vi "Check Admin Identity.vi"(8 "error in (no error)":errorcluster, 10 "UserName(\"\")":string, 11 "User_Actor in":refnum<class "User_Actor.lvclass">) -> (0 "error out":errorcluster, 2 "Identity（False）":bool, 3 "User_Actor out":refnum<class "User_Actor.lvclass">)   [LabVIEW 2015, in "User_Actor.lvlib" / "User_Actor.lvclass"]
uses:
  User_Actor.lvclass
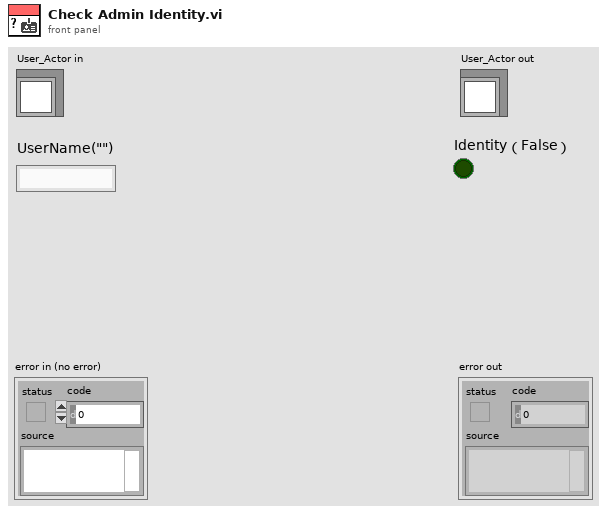
[diagram p1: front panel]
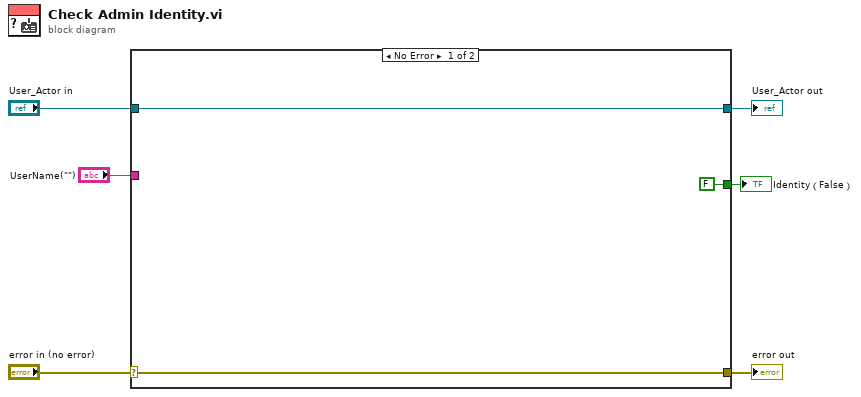
[diagram p0: block diagram]
diagram:
  n1 = case shown="No Error" "error in (no error)" {
    selector: "error in (no error)" -> [w9 w11]
    tunnel: [w9 w11] -> w5
    tunnel: [w8 w10] -> w3
    tunnel: "User_Actor in" -> [w8 w10]
    tunnel: "UserName(\"\")" -> [_ _]
    tunnel: [FALSE _] -> w1
    frame No Error {
    }
    frame Error {
    }
  }
  "error out" <- w5
  "User_Actor out" <- w3
  "Identity（False）" <- w1
